vi "ShooterDistanceCalibration.vi"(11 "Detected Totes":T1(array[cluster])) -> (2 "bottomFlyWheelConstant":dbl, 3 "TopFlyWheelConstant":dbl)   [LabVIEW 2015]
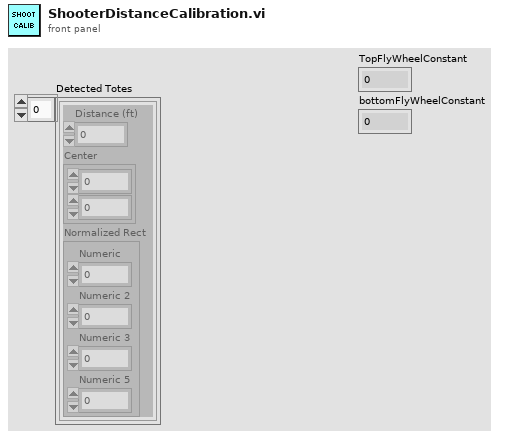
[diagram p1: front panel]
types:
  T1 = cluster{"Distance (ft)":dbl, "Center":cluster{dbl, dbl}, "Normalized Rect":cluster{"Numeric":dbl, "Numeric 2":dbl, "Numeric 3":dbl, "Numeric 5":dbl}}[]
  T2 = cluster{"Distance (ft)":dbl, "Center":cluster{dbl, dbl}, "Normalized Rect":cluster{"Numeric":dbl, "Numeric 2":dbl, "Numeric 3":dbl, "Numeric 5":dbl}}
  T3 = typedef "constants.ctl" = cluster{"motorConstants":cluster{"leftDriveMotor":u8, "rightDriveMotor":u8, "climberWinch":T4, "shooterTopFlyWheel":T4, "shooterBottomFlyWheel":T4, "climberExtender":T4, "shooterIntakeWheel":u8, "Front Arm Motor":u8}, "arduinoInputChannel":cluster{"armAngleUp":i32, "intakeWheelSpinIn":i32, "winchUp":i32, "extenderUp":i32, "AimingAuto":i32, "extenderDown":i32, "FrontArmAxis":i32, "shooter up/down":i32}, "driveConstants":cluster{"firstIntervalPercent":dbl, "secondIntervalPercent":dbl, "thirdIntervalPercent":dbl}, "cRioInputChanels":cluster{"photoEye":i32, "limitExtender":i32}, "pneumaticsChannels":cluster{"angleSolenoid":T5, "shooterAnglerPneumaticForward":T5, "shooterAnglerPneumaticReverse":T5, "Pneumatics Control Module":u8}, "flyWheelConstants":cluster{"manualTopWheel":dbl, "manualBottomWheel":dbl, "autoFuncConst1":dbl, "autoFuncConst2":dbl, "autoFuncConst3":dbl, "autoFuncConst4":dbl, "Array":dbl[][]}}
  T4 = typedef "FPGA_DIOPWMChannel.ctl" = enum8{"PWM 0", "PWM 1", "PWM 2", "PWM 3", "PWM 4", "PWM 5", "PWM 6", "PWM 7", "PWM 8", "PWM 9", "PWM MXP 0", "PWM MXP 1", "PWM MXP 2", "PWM MXP 3", "PWM MXP 4", "PWM MXP 5", "PWM MXP 6", "PWM MXP 7", "PWM MXP 8", "PWM MXP 9", "Invalid"}
  T5 = typedef "WPI_SolenoidChannel.ctl" = enum8{"Solenoid 0", "Solenoid 1", "Solenoid 2", "Solenoid 3", "Solenoid 4", "Solenoid 5", "Solenoid 6", "Solenoid 7", "Invalid"}
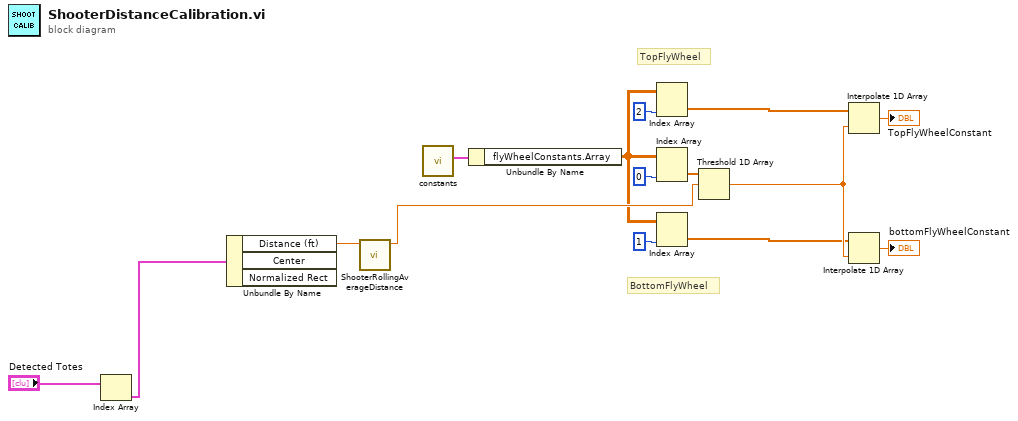
[diagram p0: block diagram]
diagram:
  # "TopFlyWheel"
  # "BottomFlyWheel"
  n1 = Index Array(array="Detected Totes") -> (element=w15:T2)  [unwired: 1 in]
  n2 = Unbundle By Name(w15) -> ("Distance (ft)"=w13:dbl)  [unwired: 2 out]
  n3 = call "ShooterRollingAverageDistance.vi"("Distance (ft)"=w13) -> ("distanceMean"=w10:dbl)  [unwired: 10 in]
  n4 = call "constants.vi"() -> (2:w12:T3)  [unwired: 11 in]
  n5 = Unbundle By Name(w12) -> ("flyWheelConstants.Array"=w8:dbl[][])
  n6 = Index Array(array=w8, index (col)=2 ("disabled index (col)")) -> (element=w4:dbl[])  [unwired: 1 in]
  n7 = Index Array(array=w8, index (col)=0 ("disabled index (col)")) -> (element=w11:dbl[])  [unwired: 1 in]
  n8 = Index Array(array=w8, index (col)=1 ("disabled index (col)")) -> (element=w3:dbl[])  [unwired: 1 in]
  n9 = Threshold 1D Array(2:w10, 3:w11) -> (0:w9:dbl)  [unwired: 1 in]
  n10 = Interpolate 1D Array(1:w9, 2:w4) -> (0:→"TopFlyWheelConstant":dbl)
  n11 = Interpolate 1D Array(1:w9, 2:w3) -> (0:→"bottomFlyWheelConstant":dbl)
